vi "DriveAngleH.vi"(3 "Parameter String":string, 4 "Reinit":bool, 5 "Auto Test Heading In (deg)":dbl) -> (0 "Error Out":errorcluster, 1 "Increment":bool, 2 "Auto Test Heading Out (deg)":dbl)   [LabVIEW 2019]
doc: "The swerve drive base will rotate about its center at a speed specified by the joystick command. This is a \"dumb\" algorithm, there is no feedback controller and the direction of rotation must be specified manually. Any complex or critical turns should be handled using either the Path Follower or auto-targeting. \n\nParameters:\n1. field-centric angle --> (deg) [0,360]\n2. relative rotation speed --> [-1,1]"
uses:
  SafeParser_Float.vi
  dsinstructions.vi
  sensors.vi
  dsdata.vi
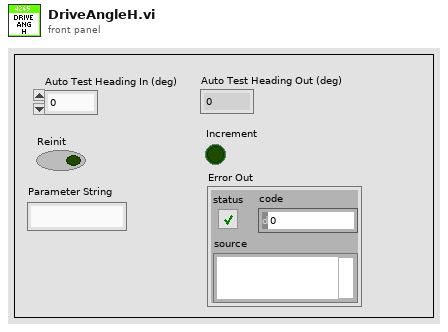
[diagram p1: front panel]
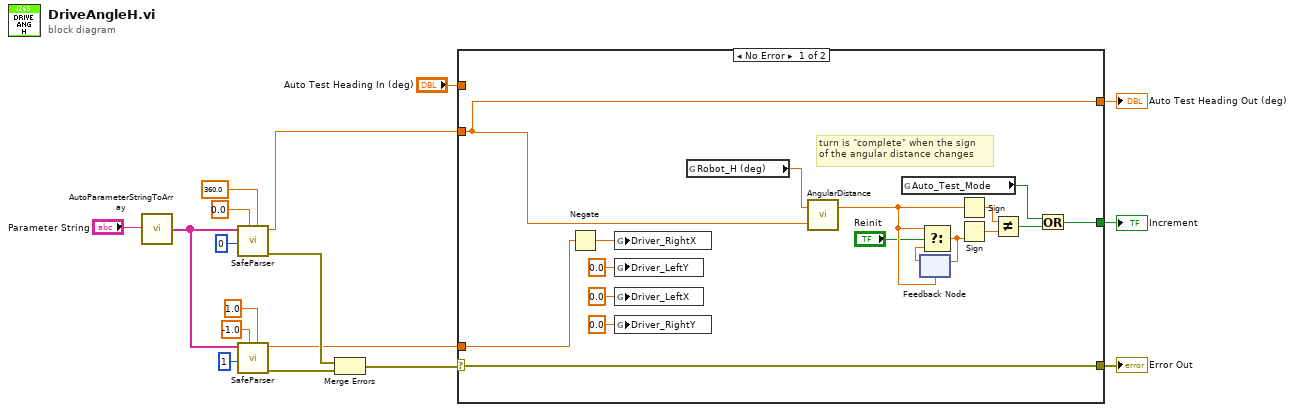
[diagram p0: block diagram]
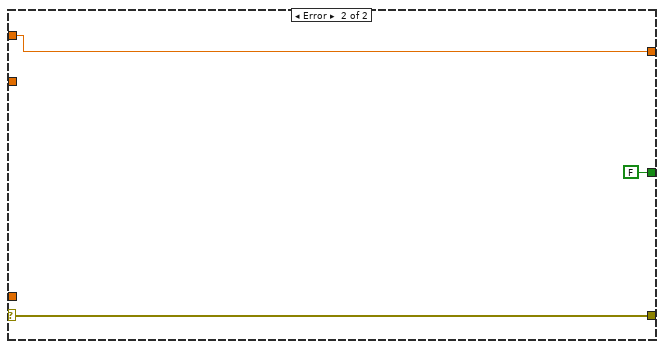
[diagram p2: hidden frame]
diagram:
  n1 = call "AutoParameterStringToArray.vi"("Parameter String"="Parameter String") -> ("Parsed Parameters"=w8:string[])
  n2 = call-poly "SafeParser.vi"("Maximum"=360.0, "Minimum"=0.0, "Array Index"=0 ("Parameter Index"), "String Array"=w8) -> ("Error Out"=w6:errorcluster, "Typecast  Value"=w4:dbl)  [unwired: 6 in]
  n3 = call-poly "SafeParser.vi"("Maximum"=1.0, "Minimum"=-1.0, "Array Index"=1 ("Parameter Index"), "String Array"=w8) -> ("Error Out"=w5:errorcluster, "Typecast  Value"=w3:dbl)  [unwired: 6 in]
  n4 = Merge Errors(w6, w5) -> (w7:errorcluster)
  n5 = case shown="No Error" w7 {
    selector: w7 -> [w24 w37]
    tunnel: [w19 FALSE] -> w17
    tunnel: [w24 w37] -> w16
    tunnel: [w22 w35] -> w15
    tunnel: "Auto Test Heading In (deg)" -> [_ w35]
    tunnel: w4 -> [w22 _]
    tunnel: w3 -> [w23 _]
    frame No Error {
      # "turn is \"complete\" when the sign\nof the angular distance changes"
      n6 = Negate(x=w23) -> (-x=w31:dbl)
      n7 = global write "dsinstructions.vi" "Driver_RightX"(w31) -> ()
      n8 = global write "dsinstructions.vi" "Driver_LeftY"(0.0 ("Driver_RightX")) -> ()
      n9 = global write "dsinstructions.vi" "Driver_LeftX"(0.0 ("Driver_RightX")) -> ()
      n10 = global write "dsinstructions.vi" "Driver_RightY"(0.0 ("Driver_RightX")) -> ()
      n11 = global read "sensors.vi" "Robot_H (deg)"() -> (w18:dbl)
      n12 = call "AngularDistance.vi"("Goal Angle (deg) [0,360]"=w22, "Current Angle (deg) [-Inf,+Inf]"=w18) -> ("Signed Angular Distance (deg) [-180,+180]"=w28:dbl)  [unwired: 1 out]
      n13 = global read "dsdata.vi" "Auto_Test_Mode"() -> (w21:bool)
      n14 = feedback #1(w28) -> (w29:dbl)
      n15 = Select(t=w28, s="Reinit", f=w29) -> (s? t:f=w30:dbl)
      n16 = feedback-in #1(w30) -> ()
      n17 = Sign(1:w28) -> (0:w26:dbl)
      n18 = Sign(1:w30) -> (0:w27:dbl)
      n19 = Not Equal?(x=w26, y=w27) -> (x != y?=w20:bool)
      n20 = Or(x=w21, y=w20) -> (x .or. y?=w19:bool)
    }
    frame Error {
    }
  }
  "Increment" <- w17
  "Auto Test Heading Out (deg)" <- w15
  "Error Out" <- w16
